vi "_Validate Calibration Table.vi"(2 "error in (no error)":errorcluster, 3 "Calibration In":dbl[][](array[numeric])) -> (0 "error out":errorcluster, 1 "Calibration Out":dbl[][](array[numeric]))   [LabVIEW 2015]
uses:
  _RT Global.vi
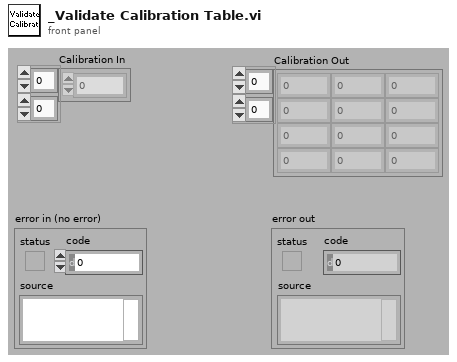
[diagram p1: front panel]
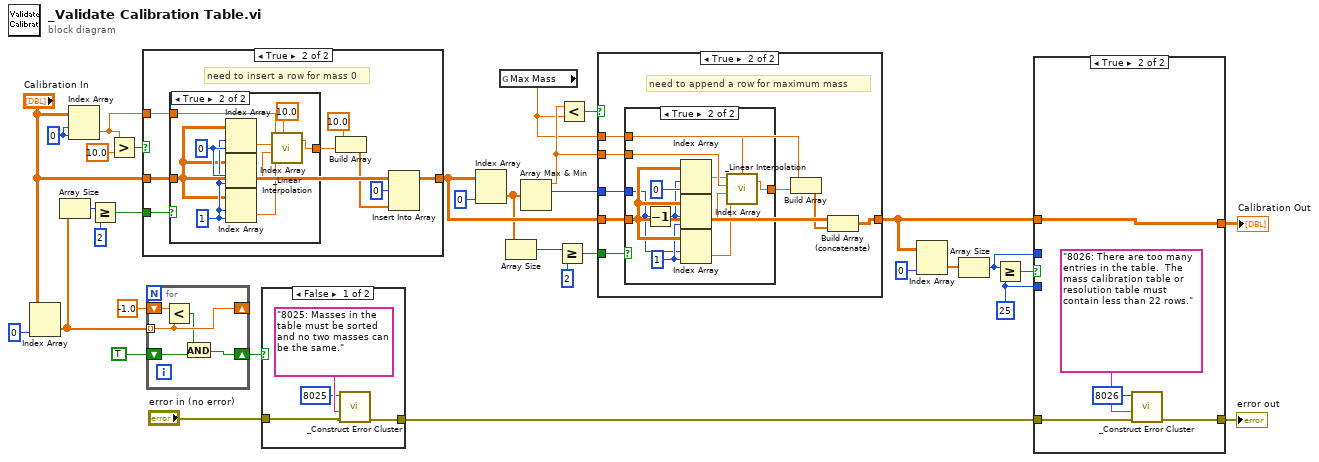
[diagram p0: block diagram]
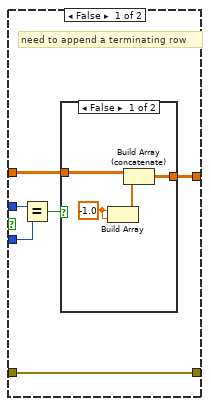
[diagram p2: hidden frame]
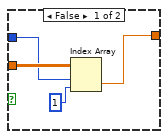
[diagram p5: hidden frame]
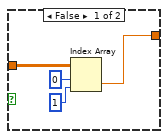
[diagram p8: hidden frame]
diagram:
  w4 = 25 ("y")
  w31 = 0 ("disabled index (row)")
  n1 = Index Array(array="Calibration In", index (col)=0 ("disabled index (row)")) -> (element=w24:dbl[])  [unwired: 1 in]
  n2 = Array Size(array=w24) -> (size(s)=w33:i32)
  n3 = Index Array(array="Calibration In", index (row)=w31, index (col)=w31) -> (element=w2:dbl)
  n4 = Greater Or Equal?(x=w33, y=2) -> (x >= y?=w23:bool)
  n5 = Greater?(x=w2, y=10.0) -> (0:w3:bool)
  n6 = case shown="True" w3 {
    tunnel: "Calibration In" -> [w34 w38]
    tunnel: w23 -> [_ w42]
    tunnel: w2 -> [_ w41]
    tunnel: [w34 w35] -> w20
    frame False {
    }
    frame True {
      # "need to insert a row for mass 0"
      n7 = case shown="True" w42 {
        tunnel: w38 -> [w45 w53]
        tunnel: w41 -> [_ w52]
        tunnel: [w43 w48] -> w39
        frame False {
          n8 = Index Array(array=w45, index (row)=0 ("disabled index (row)"), index (col)=1 ("disabled index (row)")) -> (element=w43:dbl)
        }
        frame True {
          w54 = 1 ("y")
          w55 = 0 ("y")
          n9 = Index Array(array=w53, index (row)=w54, index (col)=w55) -> (element=w51:dbl)
          n10 = Index Array(array=w53, index (row)=w55, index (col)=w54) -> (element=w50:dbl)
          n11 = Index Array(array=w53, index (row)=w54, index (col)=w54) -> (element=w49:dbl)
          n12 = call "_Linear Interpolation.vi"("X1"=w52, "X2"=w51, "Y1"=w50, "Y2"=w49, "X"=10.0) -> ("Y"=w48:dbl)  [unwired: 1 out]
        }
      }
      n13 = Build Array(10.0 ("Numeric"), w39) -> (w37:dbl[])
      n14 = Insert Into Array(array=w38, index (row)=0, new element=w37) -> (w35:dbl[][])  [unwired: 1 in]
    }
  }
  n15 = for {
    shift-right: [w59] -> _
    shift-left: -1.0 ("Numeric") -> [w60]
    tunnel: w24 -> [w59] mode=indexing
    shift-right: [w58] -> w26
    shift-left: TRUE -> [w56]
    n16 = Less?(x=w60, y=w59) -> (x < y?=w57:bool)
    n17 = And(x=w57, y=w56) -> (x .and. y?=w58:bool)
  }
  n18 = case shown="False" w26 {
    tunnel: "error in (no error)" -> [w64 w65]
    tunnel: [w63 w65] -> w9
    frame False {
      n19 = call "_Construct Error Cluster.vi"("error in"=w64, "reason"="8025: Masses in the table must be sorted and no two masses can be the same.", "errorCode"=8025) -> ("error out"=w63:errorcluster)  [unwired: 1 in, 3 out]
    }
    frame True {
    }
  }
  n20 = Index Array(array=w20, index (col)=0 ("disabled index (row)")) -> (element=w17:dbl[])  [unwired: 1 in]
  n21 = global read "_RT Global.vi" "Max Mass"() -> (w13:dbl)
  n22 = Array Size(array=w17) -> (size(s)=w14:i32)
  n23 = Array Max & Min(array=w17) -> (max value=w16:dbl, max index (indices)=w15:i32)  [unwired: 2 out]
  n24 = Greater Or Equal?(x=w14, y=2) -> (x >= y?=w18:bool)
  n25 = Less?(x=w16, y=w13) -> (x < y?=w21:bool)
  n26 = case shown="True" w21 {
    tunnel: w20 -> [w66 w71]
    tunnel: w18 -> [_ w74]
    tunnel: w16 -> [_ w73]
    tunnel: [w66 w70] -> w8
    tunnel: w15 -> [_ w69]
    tunnel: w13 -> [_ w68]
    frame False {
    }
    frame True {
      # "need to append a row for maximum mass"
      n27 = case shown="True" w74 {
        tunnel: w71 -> [w78 w88]
        tunnel: w73 -> [_ w81]
        tunnel: [w76 w85] -> w72
        tunnel: w69 -> [w75 w83]
        tunnel: w68 -> [_ w79]
        frame False {
          n28 = Index Array(array=w78, index (row)=w75, index (col)=1 ("disabled index (row)")) -> (element=w76:dbl)
        }
        frame True {
          w84 = 1 ("y")
          n29 = Decrement(x=w83) -> (x-1=w82:i32)
          n30 = Index Array(array=w88, index (row)=w82, index (col)=0 ("y")) -> (element=w80:dbl)
          n31 = Index Array(array=w88, index (row)=w82, index (col)=w84) -> (element=w87:dbl)
          n32 = Index Array(array=w88, index (row)=w83, index (col)=w84) -> (element=w86:dbl)
          n33 = call "_Linear Interpolation.vi"("X1"=w80, "X2"=w81, "Y1"=w87, "Y2"=w86, "X"=w79) -> ("Y"=w85:dbl)  [unwired: 1 out]
        }
      }
      n34 = Build Array(w68, w72) -> (w67:dbl[])
      n35 = Build Array (concatenate)(w71, w67) -> (w70:dbl[][])
    }
  }
  n36 = Index Array(array=w8, index (col)=0 ("disabled index (row)")) -> (element=w11:dbl[])  [unwired: 1 in]
  n37 = Array Size(array=w11) -> (size(s)=w5:i32)
  n38 = Greater Or Equal?(x=w5, y=w4) -> (x >= y?=w10:bool)
  n39 = case shown="True" w10 {
    tunnel: w9 -> [w93 w104]
    tunnel: w8 -> [w95 w102]
    tunnel: [w94 w102] -> w6
    tunnel: [w93 w103] -> w7
    tunnel: w5 -> [w92 _]
    tunnel: w4 -> [w91 _]
    frame False {
      # "need to append a terminating row"
      n40 = Equal?(x=w92, y=w91) -> (x = y?=w90:bool)
      n41 = case shown="False" w90 {
        tunnel: w95 -> [w98 w100]
        tunnel: [w96 w100] -> w94
        frame False {
          w99 = -1.0 ("Numeric")
          n42 = Build Array(w99, w99) -> (w97:dbl[])
          n43 = Build Array (concatenate)(w98, w97) -> (w96:dbl[][])
        }
        frame True {
        }
      }
    }
    frame True {
      n44 = call "_Construct Error Cluster.vi"("error in"=w104, "reason"="8026: There are too many entries in the table.  The mass calibration table or resolution table must contain less than 22 rows.", "errorCode"=8026) -> ("error out"=w103:errorcluster)  [unwired: 1 in, 3 out]
    }
  }
  "error out" <- w7
  "Calibration Out" <- w6
